vi "Checkers Settings Redirect.vi"   [LabVIEW 2014]
panel:
  # "Settings Re-director!"
  # "(If you're reading this,\nthe program is not working!)"
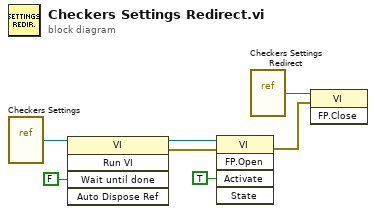
[diagram p0: block diagram]
diagram:
  n1 = vi-ref "Checkers Settings.vi"() -> (w1:refnum<vi>)
  n2 = invoke class="VI" method="Run VI"(reference=w1, "Wait until done"=FALSE ("Wait Until Done")) -> (reference out=w2:refnum<vi>, error out=w3:errorcluster)  [unwired: 3 in, 3 out]
  n3 = invoke class="VI" method="FP.Open"(reference=w2, error in=w3, "Activate"=TRUE ("Activate?")) -> (error out=w6:errorcluster)  [unwired: 2 in, 4 out]
  n4 = vi-ref "Checkers Settings Redirect.vi"() -> (w7:refnum<vi>)
  n5 = invoke class="VI" method="FP.Close"(reference=w7, error in=w6) -> ()  [unwired: 1 in, 3 out]
